vi "main.vi"() -> ()   [LabVIEW 2016]
uses:
  <vilib>/CANopenLib/CANOPEN.llb/CANopen BaudRate.ctl
  <vilib>/CANopenLib/CANOPEN.llb/CANopen Interface Create.vi
  <vilib>/CANopenLib/CANOPEN.llb/CANopen SDO Create.vi
  <vilib>/CANopenLib/CANOPEN.llb/CANopen SDO Read [I16].vi
  <vilib>/FPGAPlugInAG/cRIO-9067/niLvFpga_Open_cRIO-9067.vi
  <vilib>/rvi/interface/common/dynamic/niFpgaDynamicAddResources.vi
  <vilib>/CANopenLib/CANOPEN.llb/CANopen SDO Close.vi
  <vilib>/CANopenLib/CANOPEN.llb/CANopen Interface Close.vi
  <vilib>/FPGAPlugInAG/Dynamic/niLvFpga_Close_Dynamic.vi
  <vilib>/rvi/interface/nirviOpenFPGA/nirviOpenFPGA.xnode
  FPGA Bitfiles/CRIOCAN_FPGATarget_blank_vLBZ13piSXs.lvbitx
  <vilib>/rvi/interface/nirviCloseFPGA/nirviCloseFPGA.xnode
panel:
  out "error out":errorcluster
  in  "stop":bool
  out "I8 data":i8
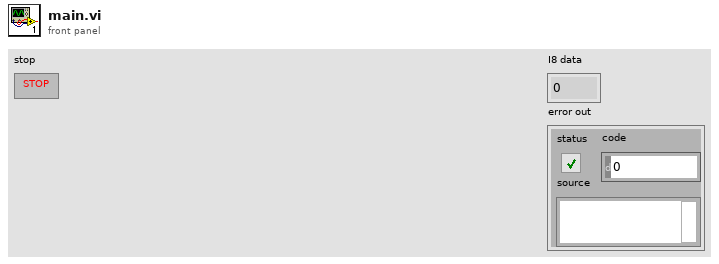
[diagram p1: front panel]
types:
  T1 = typedef "CANopen BaudRate.ctl" = u32
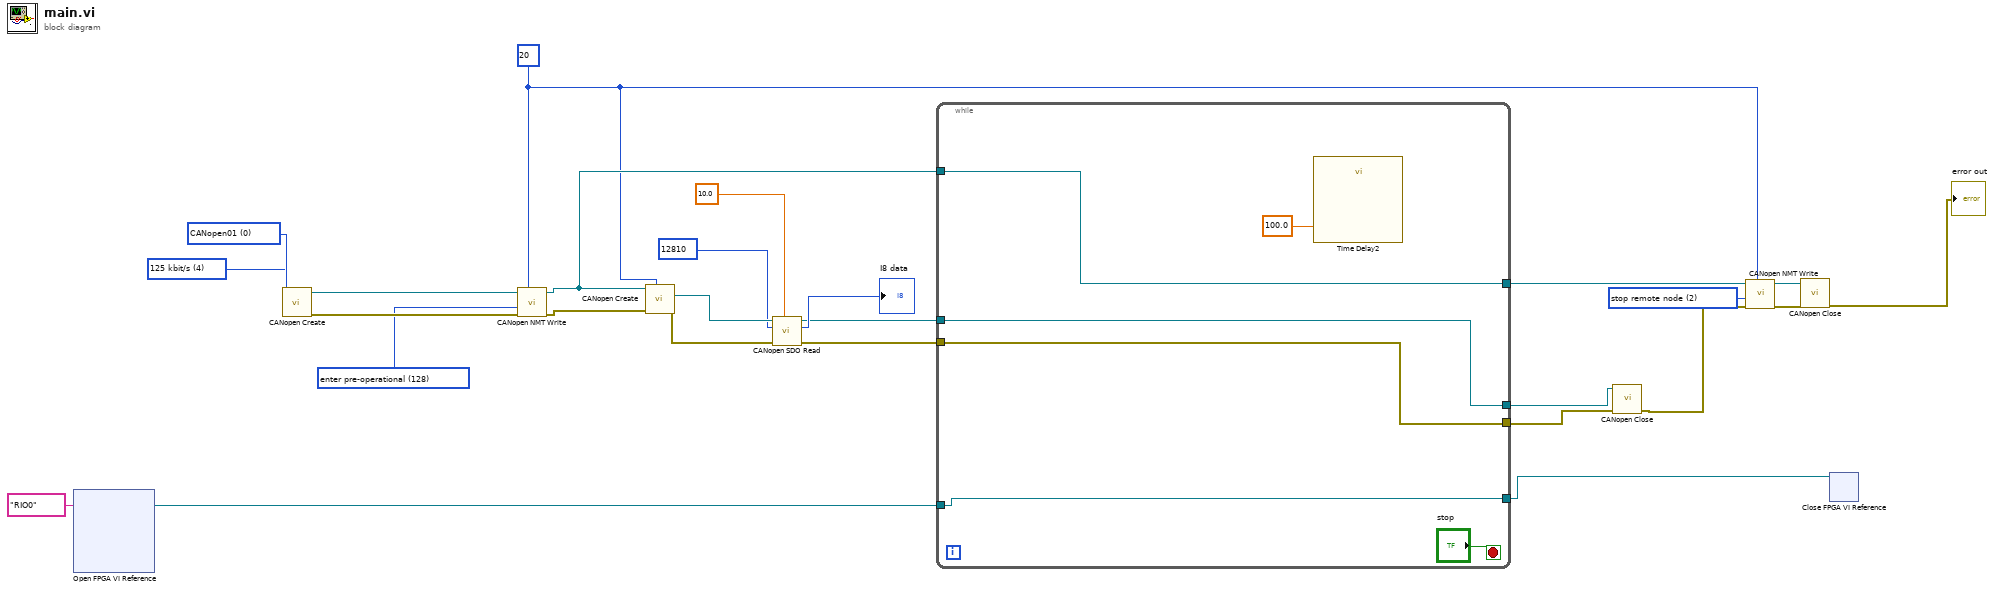
[diagram p0: block diagram]
diagram:
  w18 = u16 2 items=["start remote node"=1, "stop remote node"=2, "enter pre-operational"=128, "reset node"=129, "reset communication"=130] ("command")
  w1 = u8 20 ("node-ID (0)")
  w22 = u16 128 items=["start remote node"=1, "stop remote node"=2, "enter pre-operational"=128, "reset node"=129, "reset communication"=130] ("command")
  w25 = T1 4 items=["1 Mbit/s"=0, "800 kbit/s"=1, "500 kbit/s"=2, "250 kbit/s"=3, "125 kbit/s"=4, "50 kbit/s"=6, "20 kbit/s"=7, "10 kbit/s"=8] ("baud rate")
  w26 = u32 0 items=["CANopen01", "CANopen02", "CANopen03", "CANopen04", "CANopen05", "CANopen06", "CANopen07", "CANopen08", "CANopen09", "CANopen10", "CANopen11", "CANopen12", "CANopen13", "CANopen14", "CANopen15", "CANopen16", "CANopen17", "CANopen18", "CANopen19", "CANopen20", "CANopen21", "CANopen22", "CANopen23", "CANopen24", "CANopen25", "CANopen26", "CANopen27", "CANopen28", "CANopen29", "CANopen30", "CANopen31", "CANopen32"] ("interface name")
  n1 = xnode "Open FPGA VI Reference"("resource name"=tag "RIO0") -> ("FPGA VI Reference Out"=w15:refnum<k20>)  [unwired: 1 in, 1 out]
  n2 = call-poly <vilib>:"CANopen Create.vi"("baud rate"=w25, "interface name"=w26) -> ("error out"=w23:errorcluster, "interface object out"=w24:refnum<k20>)  [unwired: 8 in]
  n3 = call <vilib>:"CANopen NMT Write.vi"("node-ID (0)"=w1, "error in (no error)"=w23, "command"=w22, "interface object in"=w24) -> ("error out"=w12:errorcluster, "interface object out"=w4:refnum<k20>)  [unwired: 6 in]
  n4 = call-poly <vilib>:"CANopen Create.vi"("node-ID"=w1, "error in (no error)"=w12, "interface object in"=w4) -> ("error out"=w9:errorcluster, "SDO object out"=w11:refnum<k20>)  [unwired: 6 in, 1 out]
  n5 = call-poly <vilib>:"CANopen SDO Read.vi"("timeout (1s)"=10.0, "error in (no error)"=w9, "object index"=u16 12810, "SDO object in"=w11) -> ("error out"=w2:errorcluster, "I16 data"=→"I8 data":i16, "SDO object out"=w6:refnum<k20>)  [unwired: 4 in, 1 out]
  n6 = while {
    tunnel: [w28] -> w7
    tunnel: [w30] -> w14
    tunnel: w15 -> [w30]
    tunnel: w6 -> [w29]
    tunnel: [w29] -> w5
    tunnel: w4 -> [w28]
    tunnel: [w27] -> w3
    tunnel: w2 -> [w27]
    stop <- "stop" stop-if-true
    n7 = call "Time Delay2"("Delay Time (s)"=100.0) -> ()  [unwired: 10 in, 1 out]
  }
  n8 = call-poly <vilib>:"CANopen Close.vi"("error in (no error)"=w3, "SDO object in"=w5) -> ("error out"=w21:errorcluster)  [unwired: 9 in]
  n9 = call <vilib>:"CANopen NMT Write.vi"("node-ID (0)"=w1, "error in (no error)"=w21, "command"=w18, "interface object in"=w7) -> ("error out"=w20:errorcluster, "interface object out"=w19:refnum<k20>)  [unwired: 6 in]
  n10 = call-poly <vilib>:"CANopen Close.vi"("error in (no error)"=w20, "interface object in"=w19) -> ("error out"=→"error out":errorcluster)  [unwired: 9 in]
  n11 = xnode "Close FPGA VI Reference"("FPGA VI Reference In"=w14) -> ()  [unwired: 1 in, 1 out]
